vi "Assemble-camport-array.vi"(8 "error in":errorcluster, 10 "Number of cameras":i32, 11 "First camera port":enum16{"A", "B"}(ring)) -> (0 "error IO":errorcluster, 2 "Camera suffix":string[](array[string]), 3 "Camport array":u32[](array[numeric]))   [LabVIEW 2013, in "CameraVision.lvlib" / "CV-Configuration.lvclass"]
uses:
  CV-Configuration.lvclass
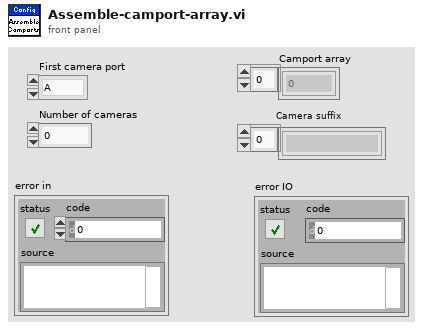
[diagram p1: front panel]
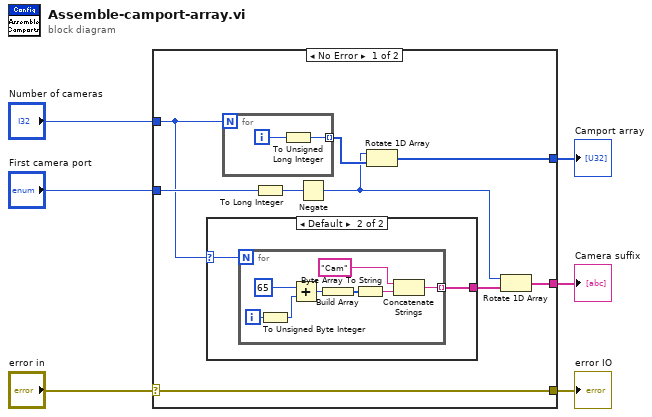
[diagram p0: block diagram]
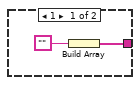
[diagram p2: hidden frame]
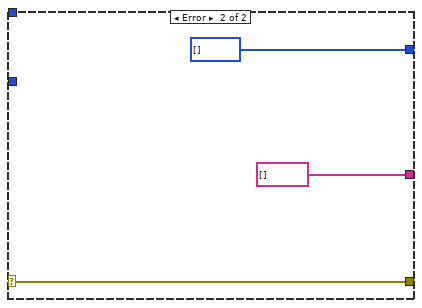
[diagram p3: hidden frame]
diagram:
  n1 = case shown="No Error" "error in" {
    selector: "error in" -> [w15 w32]
    tunnel: [w11 u32[] []] -> w6
    tunnel: "First camera port" -> [w13 _]
    tunnel: "Number of cameras" -> [w7 _]
    tunnel: [w15 w32] -> w2
    tunnel: [w9 string[] []] -> w1
    frame No Error {
      n2 = case shown="Default" w7 {
        selector: w7 -> [_ w18]
        tunnel: [w16 w19] -> w8
        frame 1 {
          n3 = Build Array("") -> (w16:string[])
        }
        frame Default {
          n4 = for {
            N: w18 -> [_]
            tunnel: [w22] -> w19 mode=indexing
            i -> [w27]
            n5 = To Unsigned Byte Integer(number=w27) -> (unsigned 8bit integer=w26:u8)
            n6 = Add(x=u8 65, y=w26) -> (x+y=w25:u8)
            n7 = Build Array(w25) -> (w24:u8[])
            n8 = Byte Array To String(unsigned byte array=w24) -> (string=w23:string)
            n9 = Concatenate Strings("Cam", w23) -> (w22:string)
          }
        }
      }
      n10 = for {
        N: w7 -> [_]
        tunnel: [w28] -> w14 mode=indexing
        i -> [w29]
        n11 = To Unsigned Long Integer(number=w29) -> (unsigned 32bit integer=w28:u32)
      }
      n12 = To Long Integer(number=w13) -> (32bit integer=w12:i32)
      n13 = Negate(x=w12) -> (-x=w10:i32)
      n14 = Rotate 1D Array(1:w14, 2:w10) -> (0:w11:u32[])
      n15 = Rotate 1D Array(1:w8, 2:w10) -> (0:w9:string[])
    }
    frame Error {
    }
  }
  "Camport array" <- w6
  "error IO" <- w2
  "Camera suffix" <- w1
